vi "Symphony Set Integration Time.vi"(0 "JYCCDLib.IJYCCDReqd":refnum<k7>, 7 "Integration (s)":dbl=10.0, 11 "Error Input":errorcluster) -> (15 "Error Output":errorcluster caption="Error Ouput")   [LabVIEW 2010]
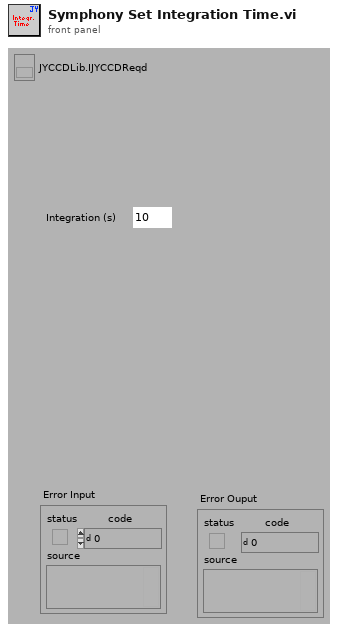
[diagram p1: front panel]
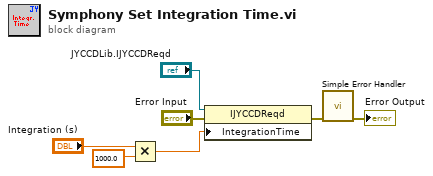
[diagram p0: block diagram]
diagram:
  n1 = Multiply(x="Integration (s)", y=1000.0) -> (x*y=w2:dbl)
  n2 = property class="IJYCCDReqd"(reference="JYCCDLib.IJYCCDReqd", error in="Error Input", "IntegrationTime"=w2) -> (error out=w1:errorcluster)  [unwired: 1 out]
  n3 = call <vilib>:"Simple Error Handler.vi"("error in (no error)"=w1) -> ("error out"=→"Error Output":errorcluster)  [unwired: 1 in, 7 out]
